vi "HGF_NetworkVisitor.appendData2Variant.vi"(0 "initData":variant, 2 "HGF_PVSubscriber":refnum<class "HGF_PVSubscriber.lvclass">, 5 "error in (no error)":errorcluster) -> (14 "dup initData":variant, 19 "error out":errorcluster)   [LabVIEW 2014, in "HGF_BaseClasses.lvlib" / "HGF_NetworkVisitor.lvclass"]
uses:
  HGF_NetworkVisitor.lvclass
  HGF_PVSubscriber/HGF_PVSubscriber.lvclass
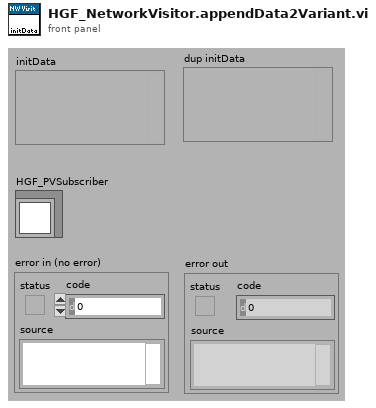
[diagram p1: front panel]
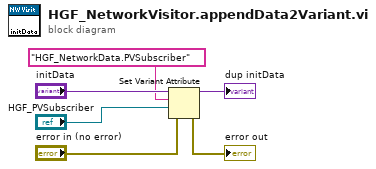
[diagram p0: block diagram]
diagram:
  n1 = Set Variant Attribute(Variant="initData", name="HGF_NetworkData.PVSubscriber", value="HGF_PVSubscriber", error in="error in (no error)") -> (Variant out=→"dup initData":variant, error out=→"error out":errorcluster)  [unwired: 1 out]
